vi "AxisMoveCtrl.vi"(9 "Home Finish":refnum<vi>, 10 "Axis":i32, 11 "PosQ":refnum<queue>) -> ()   [LabVIEW 2019]
uses:
  AxisCard.lvclass
panel:
  out "resulting string 2":string
  out "resulting string":string
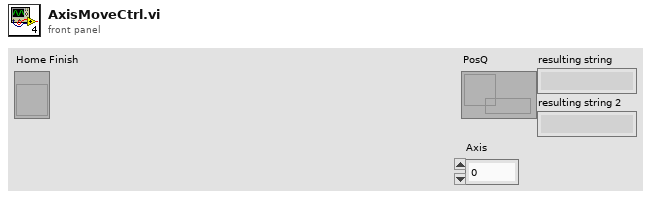
[diagram p1: front panel]
types:
  T1 = cluster{"Axis_0":bool, "Axis_1":bool, "Axis_2":bool, "Axis_3":bool, "Axis_2 2":bool, "Axis_3 2":bool}
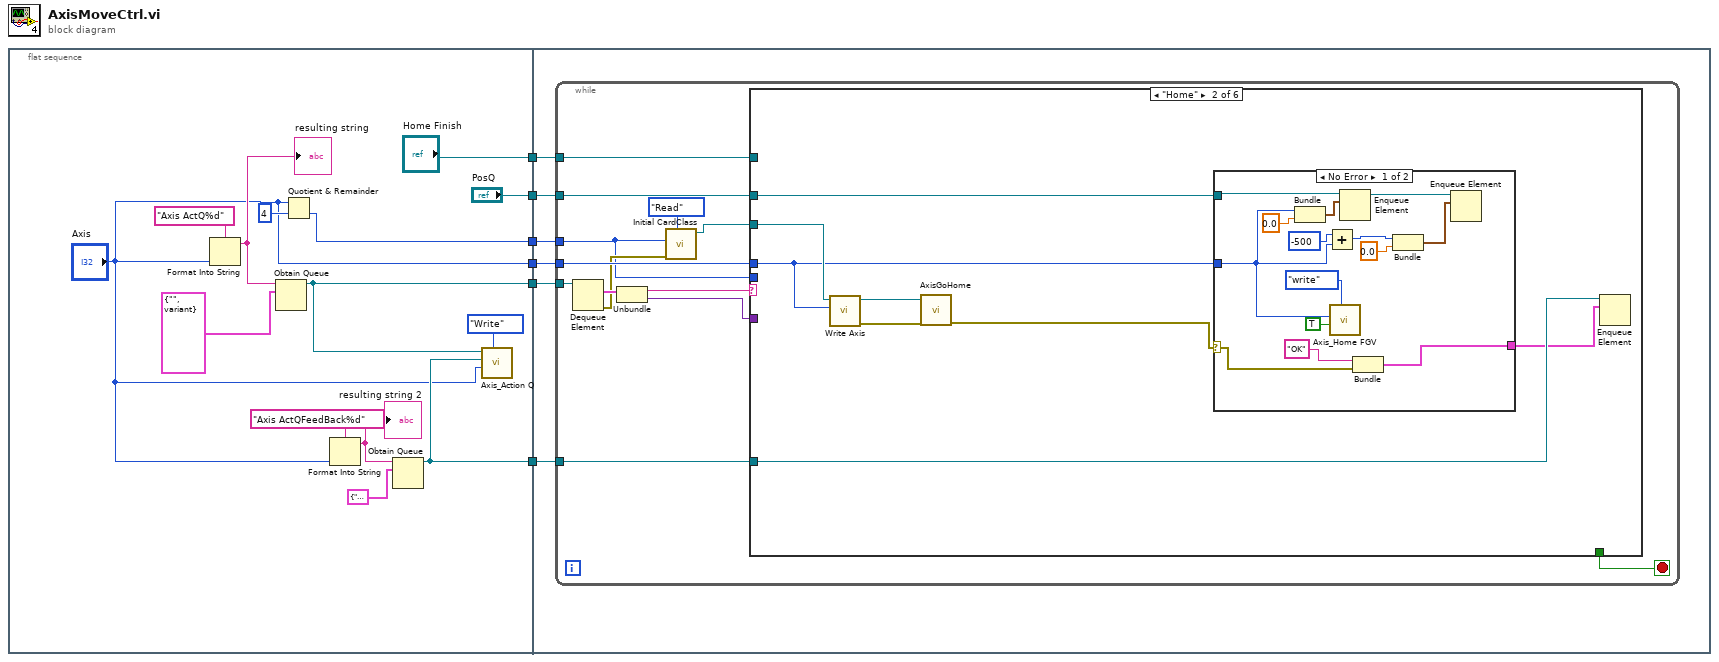
[diagram p0: block diagram]
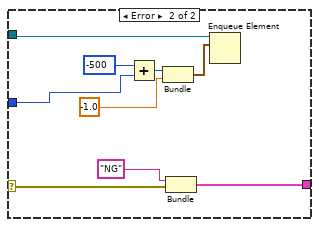
[diagram p3: hidden frame]
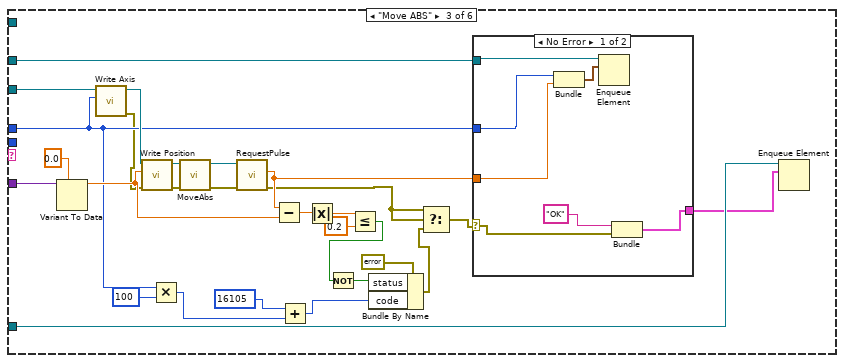
[diagram p4: hidden frame]
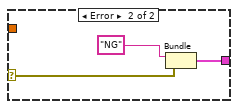
[diagram p5: hidden frame]
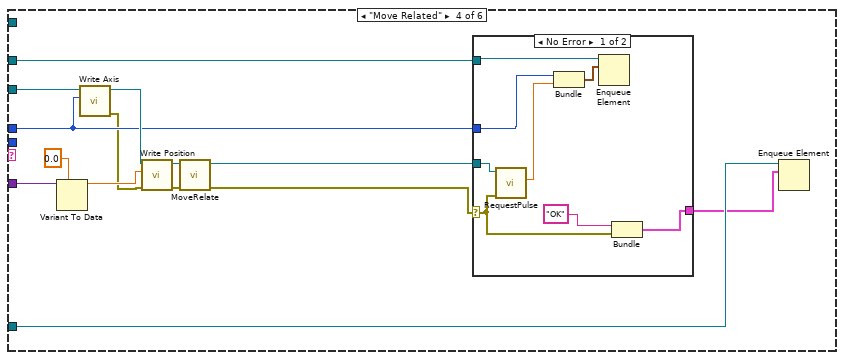
[diagram p6: hidden frame]
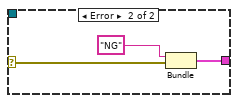
[diagram p7: hidden frame]
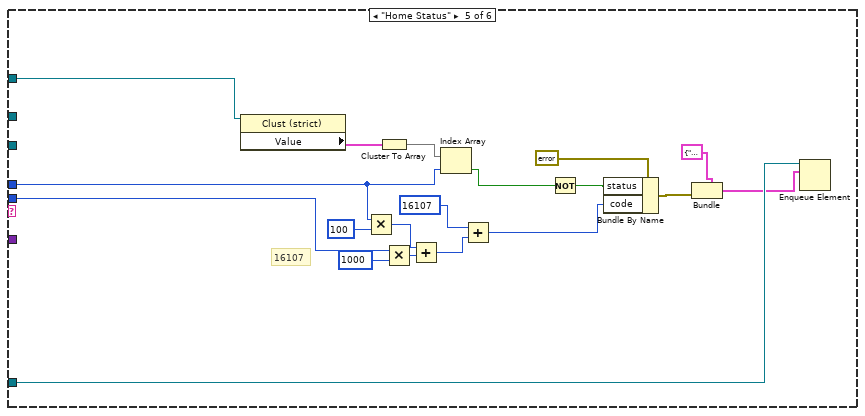
[diagram p8: hidden frame]
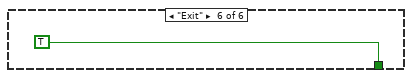
[diagram p9: hidden frame]
diagram:
  n1 = flat-sequence {
    tunnel: [w10] -> w6
    tunnel: [w9] -> w5
    tunnel: ["Axis"] -> w4
    tunnel: ["PosQ"] -> w3
    tunnel: [w12] -> w2
    tunnel: ["Home Finish"] -> w1
    tunnel: w6 -> [w26]
    tunnel: w5 -> [w25]
    tunnel: w4 -> [w24]
    tunnel: w3 -> [w23]
    tunnel: w2 -> [w22]
    tunnel: w1 -> [w21]
    frame #0 {
      n2 = Format Into String(format string="Axis ActQ%d", "Axis") -> (resulting string=w18:string)  [unwired: 2 in, 1 out]
      "resulting string" <- w18
      n3 = Obtain Queue(name (unnamed)=w18, element data type=cluster{"Action":string, "Data":variant} {"Action"="", "Data"=variant}) -> (queue out=w10:refnum<queue>)  [unwired: 3 in, 2 out]
      n4 = Quotient & Remainder(x="Axis", y=4) -> (floor(x/y)=w12:i32)  [unwired: 1 out]
      n5 = Format Into String(format string="Axis ActQFeedBack%d", "Axis") -> (resulting string=w17:string)  [unwired: 2 in, 1 out]
      "resulting string 2" <- w17
      n6 = Obtain Queue(name (unnamed)=w17, element data type=cluster{"Action":string, "Data":variant} {"Action"="", "Data"=variant}) -> (queue out=w9:refnum<queue>)  [unwired: 3 in, 2 out]
      n7 = call "Axis_Action Q.vi"("Enum"=enum16{"Initial", "Write", "Read"}."Write", "Axis Index"="Axis", "Axis ActFeedBackQ"=w9, "Axis ActQ"=w10) -> ()  [unwired: 5 in, 3 out]
    }
    frame #1 {
      n8 = while {
        tunnel: w26 -> [w39]
        tunnel: w25 -> [w35]
        tunnel: w24 -> [w34]
        tunnel: w23 -> [w33]
        tunnel: w22 -> [w27]
        tunnel: w21 -> [w28]
        stop <- w36 stop-if-true
        n9 = Dequeue Element(queue=w39) -> (element=w38:cluster{"Action":string, "Data":variant}, error out=w30:errorcluster)  [unwired: 2 in, 2 out]
        n10 = Unbundle(w38) -> ("Action"=w37:string, "Data"=w32:variant)
        n11 = call "Initial CardClass.vi"("Enum"=enum16{"Initial", "Write", "Read", "Exit"}."Read", "error in"=w30, "Card Number"=w27) -> ("DataOut"=w29:refnum<class "AxisCard.lvclass">)  [unwired: 7 in, 1 out]
        n12 = case shown="\"Home\"" w37 {
          tunnel: [_ _ _ _ _ TRUE] -> w36
          tunnel: w35 -> [_ w47 w97 w121 w152 _]
          tunnel: w29 -> [_ w43 w98 w122 _ _]
          tunnel: w34 -> [_ w42 w72 w111 w145 _]
          tunnel: w33 -> [_ w44 w95 w118 _ _]
          tunnel: w32 -> [_ _ w93 w115 _ _]
          tunnel: w28 -> [_ _ _ _ w151 _]
          tunnel: w27 -> [_ _ _ _ w148 _]
          frame "False", Default {
          }
          frame "Home" {
            n13 = call-dynamic "Write Axis.vi"("Axis"=w42, "AxisCard in"=w43) -> ("error out"=w40:errorcluster, "AxisCard out"=w41:refnum<class "AxisCard.lvclass">)  [unwired: 8 in]
            n14 = call-dynamic "AxisGoHome.vi"("error in (no error)"=w40, "AxisCard in"=w41) -> ("error out"=w46:errorcluster)  [unwired: 8 in, 1 out]
            n15 = case shown="No Error" w46 {
              selector: w46 -> [w57 w70]
              tunnel: w42 -> [w48 w65]
              tunnel: [w58 w69] -> w45
              tunnel: w44 -> [w56 w67]
              frame No Error {
                n16 = Bundle("Axis"=w48, 0.0) -> (w55:cluster{"Axis":i32, dbl})  [unwired: 1 in]
                n17 = Add(x=-500, y=w48) -> (x+y=w50:i32)
                n18 = call "Axis_Home FGV.vi"("Enum"=enum16{"Initial", "write", "read"}."write", "Home"=TRUE, "Axis"=w48) -> ()  [unwired: 7 in, 2 out]
                n19 = Enqueue Element(queue=w56, element=w55) -> (queue out=w53:refnum<queue>)  [unwired: 2 in, 2 out]
                n20 = Bundle("OK", "error IO"=w57) -> (w58:cluster{string, "error IO":errorcluster})  [unwired: 1 in]
                n21 = Bundle(w50, 0.0) -> (w52:cluster{i32, dbl})  [unwired: 1 in]
                n22 = Enqueue Element(queue=w53, element=w52) -> ()  [unwired: 2 in, 3 out]
              }
              frame Error {
                n23 = Add(x=-500 ("Axis"), y=w65) -> (x+y=w64:i32)
                n24 = Bundle(w64, "Pos"=-1.0) -> (w62:cluster{i32, "Pos":dbl})  [unwired: 1 in]
                n25 = Bundle("NG", "error IO"=w70) -> (w69:cluster{string, "error IO":errorcluster})  [unwired: 1 in]
                n26 = Enqueue Element(queue=w67, element=w62) -> ()  [unwired: 2 in, 3 out]
              }
            }
            n27 = Enqueue Element(queue=w47, element=w45) -> ()  [unwired: 2 in, 3 out]
          }
          frame "Move ABS" {
            n28 = Variant To Data(type=0.0, Variant=w93) -> (data=w87:dbl)  [unwired: 1 in, 1 out]
            n29 = call-dynamic "Write Axis.vi"("Axis"=w72, "AxisCard in"=w98) -> ("error out"=w71:errorcluster, "AxisCard out"=w73:refnum<class "AxisCard.lvclass">)  [unwired: 8 in]
            n30 = call-dynamic "Write Position.vi"("error in (no error)"=w71, "Position"=w87, "AxisCard in"=w73) -> ("error out"=w91:errorcluster, "AxisCard out"=w94:refnum<class "AxisCard.lvclass">)  [unwired: 7 in]
            n31 = Multiply(x=w72, y=100) -> (x*y=w75:i32)
            n32 = call-dynamic "MoveAbs.vi"("error in (no error)"=w91, "AxisCard in"=w94) -> ("error out"=w90:errorcluster, "AxisCard out"=w89:refnum<class "AxisCard.lvclass">)  [unwired: 8 in]
            n33 = call-dynamic "RequestPulse.vi"("error in (no error)"=w90, "AxisCard in"=w89) -> ("error out"=w83:errorcluster, "Pulse"=w88:dbl)  [unwired: 7 in, 1 out]
            n34 = Subtract(x=w88, y=w87) -> (x-y=w86:dbl)
            n35 = Add(x=16105, y=w75) -> (x+y=w77:i32)
            n36 = Absolute Value(x=w86) -> (abs(x)=w85:dbl)
            n37 = Less Or Equal?(x=w85, y=0.2) -> (x <= y?=w80:bool)
            n38 = Not(x=w80) -> (.not. x?=w81:bool)
            n39 = Bundle By Name(cluster=errorcluster {"status"=FALSE, "code"=0, "source"=""} ("error constant"), "status"=w81, "code"=w77) -> (w79:errorcluster)
            n40 = Select(t=w83, s=w83, f=w79) -> (s? t:f=w74:errorcluster)
            n41 = case shown="No Error" w74 {
              selector: w74 -> [w100 w106]
              tunnel: w72 -> [w101 _]
              tunnel: [w104 w108] -> w96
              tunnel: w95 -> [w103 _]
              tunnel: w88 -> [w99 _]
              frame No Error {
                n42 = Bundle("Axis"=w101, "Pulse"=w99) -> (w102:cluster{"Axis":i32, "Pulse":dbl})  [unwired: 1 in]
                n43 = Enqueue Element(queue=w103, element=w102) -> ()  [unwired: 2 in, 3 out]
                n44 = Bundle("OK", "error IO"=w100) -> (w104:cluster{string, "error IO":errorcluster})  [unwired: 1 in]
              }
              frame Error {
                n45 = Bundle("NG", "error IO"=w106) -> (w108:cluster{string, "error IO":errorcluster})  [unwired: 1 in]
              }
            }
            n46 = Enqueue Element(queue=w97, element=w96) -> ()  [unwired: 2 in, 3 out]
          }
          frame "Move Related" {
            n47 = Variant To Data(type=0.0, Variant=w115) -> (data=w113:dbl)  [unwired: 1 in, 1 out]
            n48 = call-dynamic "Write Axis.vi"("Axis"=w111, "AxisCard in"=w122) -> ("error out"=w109:errorcluster, "AxisCard out"=w112:refnum<class "AxisCard.lvclass">)  [unwired: 8 in]
            n49 = call-dynamic "Write Position.vi"("error in (no error)"=w109, "Position"=w113, "AxisCard in"=w112) -> ("error out"=w110:errorcluster, "AxisCard out"=w116:refnum<class "AxisCard.lvclass">)  [unwired: 7 in]
            n50 = call-dynamic "MoveRelate.vi"("error in (no error)"=w110, "AxisCard in"=w116) -> ("error out"=w120:errorcluster, "AxisCard out"=w117:refnum<class "AxisCard.lvclass">)  [unwired: 8 in]
            n51 = case shown="No Error" w120 {
              selector: w120 -> [w125 w133]
              tunnel: w111 -> [w126 _]
              tunnel: [w129 w132] -> w119
              tunnel: w118 -> [w128 _]
              tunnel: w117 -> [w124 _]
              frame No Error {
                n52 = call-dynamic "RequestPulse.vi"("error in (no error)"=w125, "AxisCard in"=w124) -> ("Pulse"=w123:dbl)  [unwired: 7 in, 2 out]
                n53 = Bundle("Axis"=w126, "Pulse"=w123) -> (w127:cluster{"Axis":i32, "Pulse":dbl})  [unwired: 1 in]
                n54 = Enqueue Element(queue=w128, element=w127) -> ()  [unwired: 2 in, 3 out]
                n55 = Bundle("OK", "error IO"=w125) -> (w129:cluster{string, "error IO":errorcluster})  [unwired: 1 in]
              }
              frame Error {
                n56 = Bundle("NG", "error IO"=w133) -> (w132:cluster{string, "error IO":errorcluster})  [unwired: 1 in]
              }
            }
            n57 = Enqueue Element(queue=w121, element=w119) -> ()  [unwired: 2 in, 3 out]
          }
          frame "Home Status" {
            # "16107"
            n58 = property class="Clust (strict)"(reference=w151) -> ("Value"=w150:T1)  [unwired: 1 in, 2 out]
            n59 = Multiply(x=w145, y=100) -> (x*y=w143:i32)
            n60 = Cluster To Array(cluster=w150) -> (array=w149:bool[])
            n61 = Multiply(x=w148, y=1000) -> (x*y=w146:i32)
            n62 = Add(x=w143, y=w146) -> (x+y=w141:i32)
            n63 = Index Array(array=w149, index=w145) -> (element=w136:bool)
            n64 = Add(x=16107, y=w141) -> (x+y=w134:i32)
            n65 = Not(x=w136) -> (.not. x?=w135:bool)
            n66 = Bundle By Name(cluster=errorcluster {"status"=FALSE, "code"=0, "source"=""} ("error constant"), "status"=w135, "code"=w134) -> (w137:errorcluster)
            n67 = Bundle(cluster=cluster{"Action":string, "Data":variant} {"Action"="", "Data"=variant} ("element"), "Data"=w137) -> (w139:cluster{"Action":string, "Data":variant})  [unwired: 1 in]
            n68 = Enqueue Element(queue=w152, element=w139) -> ()  [unwired: 2 in, 3 out]
          }
          frame "Exit" {
          }
        }
      }
    }
  }
